vi "H5Tenum_valueof.vi"   [LabVIEW 2017]
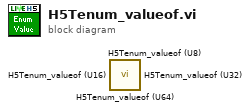
[diagram p0: block diagram]
diagram:
  n1 = call <vilib>:"H5Tenum_valueof (U64).vi"() -> ()  [unwired: 7 in, 3 out]
  n2 = call <vilib>:"H5Tenum_valueof (U8).vi"() -> ()  [unwired: 7 in, 3 out]
  n3 = call <vilib>:"H5Tenum_valueof (U16).vi"() -> ()  [unwired: 7 in, 3 out]
  n4 = call <vilib>:"H5Tenum_valueof (U32).vi"() -> ()  [unwired: 7 in, 3 out]
